vi "CallVI.lua.vi"(0 "L":u64, 1 "Lua Dll":path) -> ()   [LabVIEW 2014]
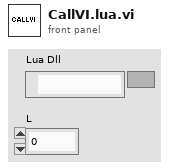
[diagram p1: front panel]
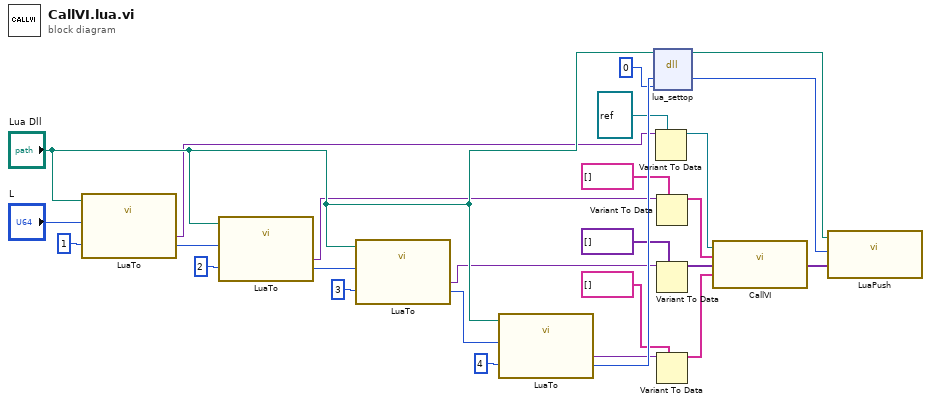
[diagram p0: block diagram]
diagram:
  n1 = call "LuaTo.vi"("Index"=1 ("n"), "L In"="L", "Lua Dll"="Lua Dll") -> ("Variant"=w14:variant, "L Out"=w19:u64)  [unwired: 4 out]
  n2 = call "LuaTo.vi"("Index"=2 ("n"), "L In"=w19, "Lua Dll"="Lua Dll") -> ("Variant"=w12:variant, "L Out"=w26:u64)  [unwired: 4 out]
  n3 = call "LuaTo.vi"("Index"=3 ("n"), "L In"=w26, "Lua Dll"="Lua Dll") -> ("Variant"=w8:variant, "L Out"=w25:u64)  [unwired: 4 out]
  n4 = call "LuaTo.vi"("Index"=4 ("n"), "L In"=w25, "Lua Dll"="Lua Dll") -> ("Variant"=w5:variant, "L Out"=w20:u64)  [unwired: 4 out]
  n5 = dll-call lib="lua5.dll" fn="lua_settop"(path in="Lua Dll", "L"=w20, "idx"=0) -> (path out=w3:path, "L"=w2:u64)  [unwired: 4 in, 1 out]
  n6 = Variant To Data(type=refnum<vi> refnum ("vi reference"), Variant=w14) -> (data=w17:refnum<vi>)  [unwired: 1 in, 1 out]
  n7 = Variant To Data(type=string[] [] ("Input Names"), Variant=w12) -> (data=w22:string[])  [unwired: 1 in, 1 out]
  n8 = Variant To Data(type=variant[] [] ("Input Values"), Variant=w8) -> (data=w23:variant[])  [unwired: 1 in, 1 out]
  n9 = Variant To Data(type=string[] [] ("Input Names"), Variant=w5) -> (data=w24:string[])  [unwired: 1 in, 1 out]
  n10 = call "CallVI.vi"("Output Names"=w24, "Input Values"=w23, "Input Names"=w22, "VI"=w17) -> ("Output Values"=w1:variant[])
  n11 = call "LuaPush.vi"("Variant"=w1, "L In"=w2, "Lua Dll"=w3) -> ()  [unwired: 1 out]
